vi "OnLine.vi"(8 "Uart Input":cluster{u64} {"?" format="%x"}, 11 "Error Input":errorcluster) -> (0 "Uart Output":cluster{u64} {"?" format="%x"}, 2 "On Line Event":refnum<event-registration>, 3 "Error Output":errorcluster)   [LabVIEW 2019]
doc: "Add an <B>On Line Received</B> event listener to the serial port."
uses:
  dll/LabViewUart.dll
panel:
  # "Add an On_Line event listenner"
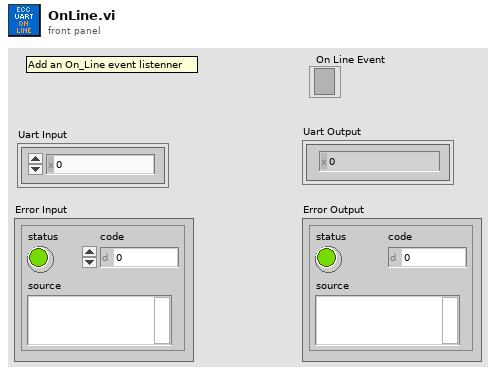
[diagram p1: front panel]
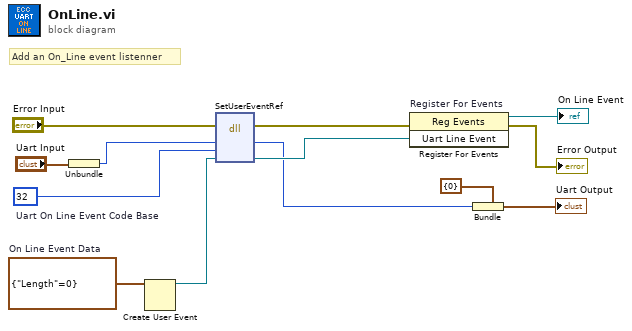
[diagram p0: block diagram]
diagram:
  w7 = cluster{"Length":u16} {"Length"=0}  # On Line Event Data
  w13 = u16 32  # Uart On Line Event Code Base
  # "Add an On_Line event listenner"
  n1 = Unbundle("Uart Input") -> (w1:u64)
  n2 = Create User Event(user event datatype=w7) -> (user event=w11:refnum<user-event>)  [unwired: 1 in, 1 out]
  n3 = dll-call lib="D:/Google Drive/INC-2020/INC352/INC352-2020/LabVIEW/examples/uart-cmdex/SubVI/dll/LabViewUart.dll" fn="SetUserEventRef"(error in="Error Input", "Uart Handle"=w1, "Uart On Line Event Code Base"=w13, "Uart Line Event"=w11) -> (error out=w9:errorcluster, "Uart Handle"=w3:u64, "Uart Line Event"=w12:refnum<user-event>)  [unwired: 4 in, 1 out]
  n4 = register-events "Register For Events"(error in=w9, w12) -> (reference out=→"On Line Event":refnum<event-registration>, error out=→"Error Output":errorcluster)  [unwired: 1 in]
  n5 = Bundle(cluster=cluster{u64} {0}, w3) -> (→"Uart Output":cluster{u64})
